vi "Set Controls Enable or Disable State.vi"(8 "error in (no error)":errorcluster, 10 "Refnum State":T2=enum."Start Live", 11 "Refnums In":T1) -> (0 "error out":errorcluster)   [LabVIEW 2017]
uses:
  Controls/Enabled State Control.ctl
  Controls/Refnums.ctl
  Controls/Recording Settings.ctl
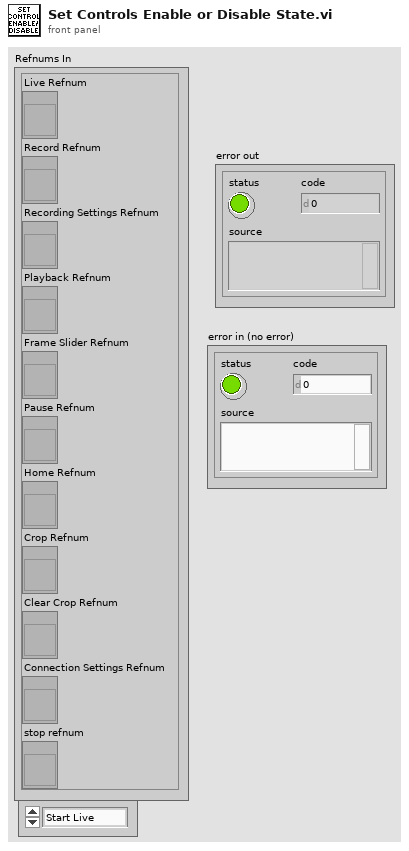
[diagram p1: front panel]
types:
  T1 = typedef "Refnums.ctl" = cluster{"Live Refnum":refnum<vi>, "Record Refnum":refnum<vi>, "Recording Settings Refnum":refnum<vi>, "Playback Refnum":refnum<vi>, "Frame Slider Refnum":refnum<vi>, "Pause Refnum":refnum<vi>, "Home Refnum":refnum<vi>, "Crop Refnum":refnum<vi>, "Clear Crop Refnum":refnum<vi>, "Connection Settings Refnum":refnum<vi>, "stop refnum":refnum<vi>}
  T2 = typedef "Enabled State Control.ctl" = enum16{"Wait", "Start Live", "Start Recording", "Start Playback", "Shutdown"}
  T3 = enum8{"Enabled", "Disabled", "Disabled and Grayed Out"}
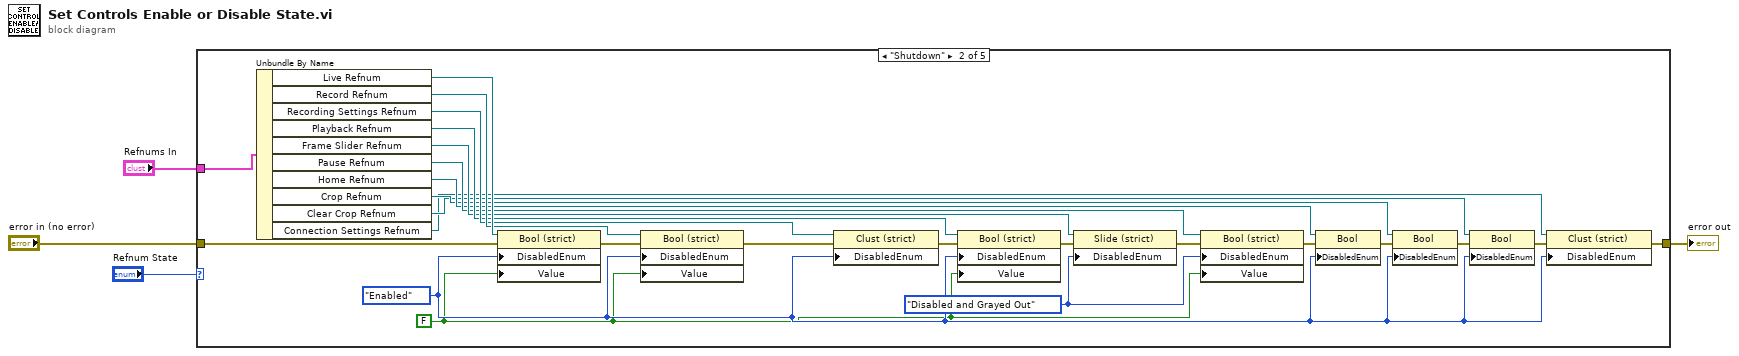
[diagram p0: block diagram]
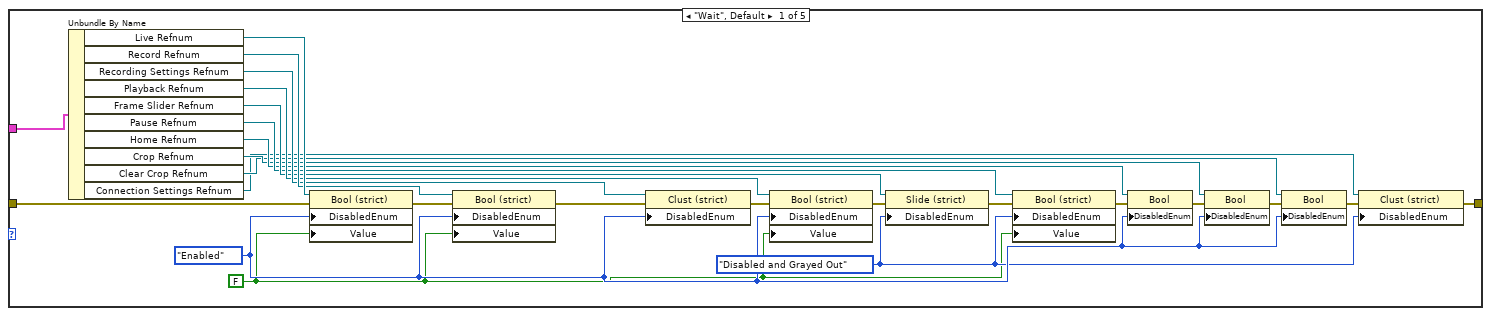
[diagram p2: hidden frame]
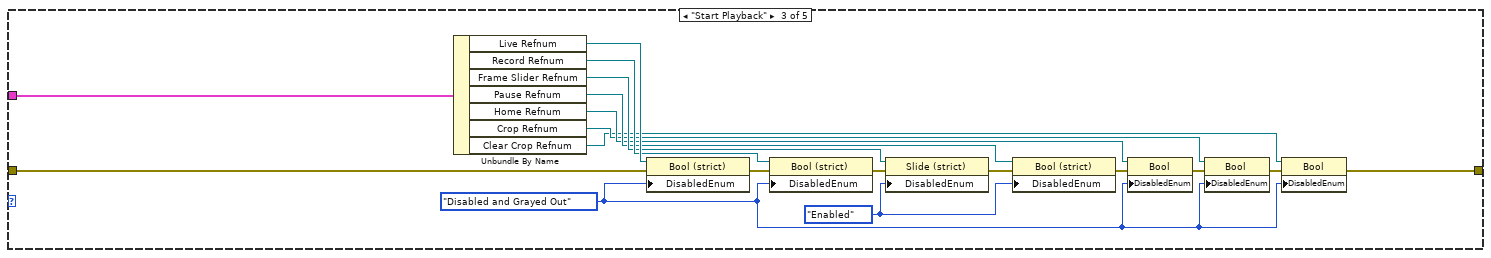
[diagram p3: hidden frame]
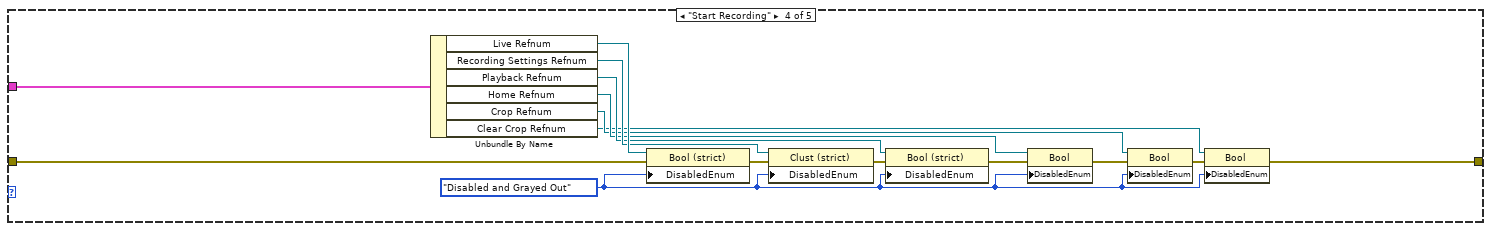
[diagram p4: hidden frame]
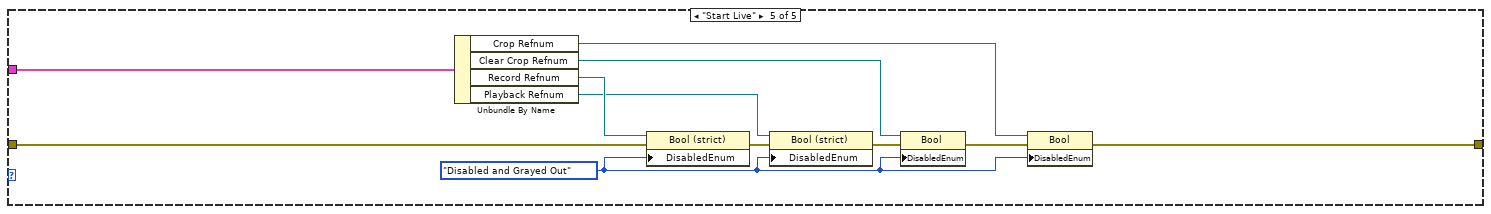
[diagram p5: hidden frame]
diagram:
  n1 = case shown="\"Shutdown\"" "Refnum State" {
    tunnel: "Refnums In" -> [w29 w54 w72 w87 w98]
    tunnel: "error in (no error)" -> [w18 w44 w64 w80 w94]
    tunnel: [w8 w33 w56 w74 w89] -> w4
    frame "Wait", Default {
      w5 = FALSE
      w9 = T3."Disabled and Grayed Out" ("Disabled")
      w19 = T3."Enabled" ("Disabled")
      n2 = Unbundle By Name(w29) -> ("Live Refnum"=w28:refnum<vi>, "Record Refnum"=w27:refnum<vi>, "Recording Settings Refnum"=w26:refnum<vi>, "Playback Refnum"=w25:refnum<vi>, "Frame Slider Refnum"=w24:refnum<vi>, "Pause Refnum"=w23:refnum<vi>, "Home Refnum"=w22:refnum<vi>, "Crop Refnum"=w21:refnum<vi>, "Clear Crop Refnum"=w20:refnum<vi>, "Connection Settings Refnum"=w7:refnum<vi>)
      n3 = property class="Bool (strict)"(reference=w28, error in=w18, "DisabledEnum"=w19, "Value"=w5) -> (error out=w17:errorcluster)  [unwired: 1 out]
      n4 = property class="Bool (strict)"(reference=w27, error in=w17, "DisabledEnum"=w19, "Value"=w5) -> (error out=w16:errorcluster)  [unwired: 1 out]
      n5 = property class="Clust (strict)"(reference=w26, error in=w16, "DisabledEnum"=w19) -> (error out=w15:errorcluster)  [unwired: 1 out]
      n6 = property class="Bool (strict)"(reference=w25, error in=w15, "DisabledEnum"=w19, "Value"=w5) -> (error out=w14:errorcluster)  [unwired: 1 out]
      n7 = property class="Slide (strict)"(reference=w24, error in=w14, "DisabledEnum"=w9) -> (error out=w13:errorcluster)  [unwired: 1 out]
      n8 = property class="Bool (strict)"(reference=w23, error in=w13, "DisabledEnum"=w9, "Value"=w5) -> (error out=w12:errorcluster)  [unwired: 1 out]
      n9 = property class="Bool"(reference=w22, error in=w12, "DisabledEnum"=w19) -> (error out=w11:errorcluster)  [unwired: 1 out]
      n10 = property class="Bool"(reference=w21, error in=w11, "DisabledEnum"=w19) -> (error out=w10:errorcluster)  [unwired: 1 out]
      n11 = property class="Bool"(reference=w20, error in=w10, "DisabledEnum"=w19) -> (error out=w6:errorcluster)  [unwired: 1 out]
      n12 = property class="Clust (strict)"(reference=w7, error in=w6, "DisabledEnum"=w9) -> (error out=w8:errorcluster)  [unwired: 1 out]
    }
    frame "Shutdown" {
      w30 = FALSE
      w32 = T3."Disabled and Grayed Out" ("Disabled")
      w31 = T3."Enabled" ("Disabled")
      n13 = Unbundle By Name(w54) -> ("Live Refnum"=w53:refnum<vi>, "Record Refnum"=w52:refnum<vi>, "Recording Settings Refnum"=w51:refnum<vi>, "Playback Refnum"=w50:refnum<vi>, "Frame Slider Refnum"=w49:refnum<vi>, "Pause Refnum"=w48:refnum<vi>, "Home Refnum"=w47:refnum<vi>, "Crop Refnum"=w46:refnum<vi>, "Clear Crop Refnum"=w45:refnum<vi>, "Connection Settings Refnum"=w35:refnum<vi>)
      n14 = property class="Bool (strict)"(reference=w53, error in=w44, "DisabledEnum"=w31, "Value"=w30) -> (error out=w43:errorcluster)  [unwired: 1 out]
      n15 = property class="Bool (strict)"(reference=w52, error in=w43, "DisabledEnum"=w31, "Value"=w30) -> (error out=w42:errorcluster)  [unwired: 1 out]
      n16 = property class="Clust (strict)"(reference=w51, error in=w42, "DisabledEnum"=w31) -> (error out=w41:errorcluster)  [unwired: 1 out]
      n17 = property class="Bool (strict)"(reference=w50, error in=w41, "DisabledEnum"=w31, "Value"=w30) -> (error out=w40:errorcluster)  [unwired: 1 out]
      n18 = property class="Slide (strict)"(reference=w49, error in=w40, "DisabledEnum"=w32) -> (error out=w39:errorcluster)  [unwired: 1 out]
      n19 = property class="Bool (strict)"(reference=w48, error in=w39, "DisabledEnum"=w32, "Value"=w30) -> (error out=w38:errorcluster)  [unwired: 1 out]
      n20 = property class="Bool"(reference=w47, error in=w38, "DisabledEnum"=w31) -> (error out=w37:errorcluster)  [unwired: 1 out]
      n21 = property class="Bool"(reference=w46, error in=w37, "DisabledEnum"=w31) -> (error out=w36:errorcluster)  [unwired: 1 out]
      n22 = property class="Bool"(reference=w45, error in=w36, "DisabledEnum"=w31) -> (error out=w34:errorcluster)  [unwired: 1 out]
      n23 = property class="Clust (strict)"(reference=w35, error in=w34, "DisabledEnum"=w31) -> (error out=w33:errorcluster)  [unwired: 1 out]
    }
    frame "Start Playback" {
      w57 = T3."Disabled and Grayed Out" ("Disabled")
      w58 = T3."Enabled" ("Disabled")
      n24 = Unbundle By Name(w72) -> ("Live Refnum"=w71:refnum<vi>, "Record Refnum"=w70:refnum<vi>, "Frame Slider Refnum"=w69:refnum<vi>, "Pause Refnum"=w68:refnum<vi>, "Home Refnum"=w67:refnum<vi>, "Crop Refnum"=w66:refnum<vi>, "Clear Crop Refnum"=w65:refnum<vi>)
      n25 = property class="Bool (strict)"(reference=w71, error in=w64, "DisabledEnum"=w57) -> (error out=w63:errorcluster)  [unwired: 1 out]
      n26 = property class="Bool (strict)"(reference=w70, error in=w63, "DisabledEnum"=w57) -> (error out=w55:errorcluster)  [unwired: 1 out]
      n27 = property class="Slide (strict)"(reference=w69, error in=w55, "DisabledEnum"=w58) -> (error out=w62:errorcluster)  [unwired: 1 out]
      n28 = property class="Bool (strict)"(reference=w68, error in=w62, "DisabledEnum"=w58) -> (error out=w61:errorcluster)  [unwired: 1 out]
      n29 = property class="Bool"(reference=w67, error in=w61, "DisabledEnum"=w57) -> (error out=w60:errorcluster)  [unwired: 1 out]
      n30 = property class="Bool"(reference=w66, error in=w60, "DisabledEnum"=w57) -> (error out=w59:errorcluster)  [unwired: 1 out]
      n31 = property class="Bool"(reference=w65, error in=w59, "DisabledEnum"=w57) -> (error out=w56:errorcluster)  [unwired: 1 out]
    }
    frame "Start Recording" {
      w75 = T3."Disabled and Grayed Out" ("Disabled")
      n32 = Unbundle By Name(w87) -> ("Live Refnum"=w86:refnum<vi>, "Recording Settings Refnum"=w85:refnum<vi>, "Playback Refnum"=w84:refnum<vi>, "Home Refnum"=w83:refnum<vi>, "Crop Refnum"=w82:refnum<vi>, "Clear Crop Refnum"=w81:refnum<vi>)
      n33 = property class="Bool (strict)"(reference=w86, error in=w80, "DisabledEnum"=w75) -> (error out=w76:errorcluster)  [unwired: 1 out]
      n34 = property class="Clust (strict)"(reference=w85, error in=w76, "DisabledEnum"=w75) -> (error out=w79:errorcluster)  [unwired: 1 out]
      n35 = property class="Bool (strict)"(reference=w84, error in=w79, "DisabledEnum"=w75) -> (error out=w73:errorcluster)  [unwired: 1 out]
      n36 = property class="Bool"(reference=w83, error in=w73, "DisabledEnum"=w75) -> (error out=w78:errorcluster)  [unwired: 1 out]
      n37 = property class="Bool"(reference=w82, error in=w78, "DisabledEnum"=w75) -> (error out=w77:errorcluster)  [unwired: 1 out]
      n38 = property class="Bool"(reference=w81, error in=w77, "DisabledEnum"=w75) -> (error out=w74:errorcluster)  [unwired: 1 out]
    }
    frame "Start Live" {
      w88 = T3."Disabled and Grayed Out" ("Disabled")
      n39 = Unbundle By Name(w98) -> ("Crop Refnum"=w93:refnum<vi>, "Clear Crop Refnum"=w92:refnum<vi>, "Record Refnum"=w97:refnum<vi>, "Playback Refnum"=w96:refnum<vi>)
      n40 = property class="Bool (strict)"(reference=w97, error in=w94, "DisabledEnum"=w88) -> (error out=w95:errorcluster)  [unwired: 1 out]
      n41 = property class="Bool (strict)"(reference=w96, error in=w95, "DisabledEnum"=w88) -> (error out=w91:errorcluster)  [unwired: 1 out]
      n42 = property class="Bool"(reference=w92, error in=w91, "DisabledEnum"=w88) -> (error out=w90:errorcluster)  [unwired: 1 out]
      n43 = property class="Bool"(reference=w93, error in=w90, "DisabledEnum"=w88) -> (error out=w89:errorcluster)  [unwired: 1 out]
    }
  }
  "error out" <- w4
